vi "Read RT Variables.vi"(8 "error in (no error)":errorcluster, 11 "functionbase in":refnum<class "functionbase.lvclass">) -> (0 "error out":errorcluster, 2 "RT Variables.lvclass":refnum<class "RT Variables.lvclass">, 3 "functionbase out":refnum<class "functionbase.lvclass">)   [LabVIEW 2019, in "LSL.lvlib" / "functionbase.lvclass"]
uses:
  functionbase.lvclass
  variables/RT Variables/RT Variables.lvclass
  functionbase.lvclass/functionbase.ctl
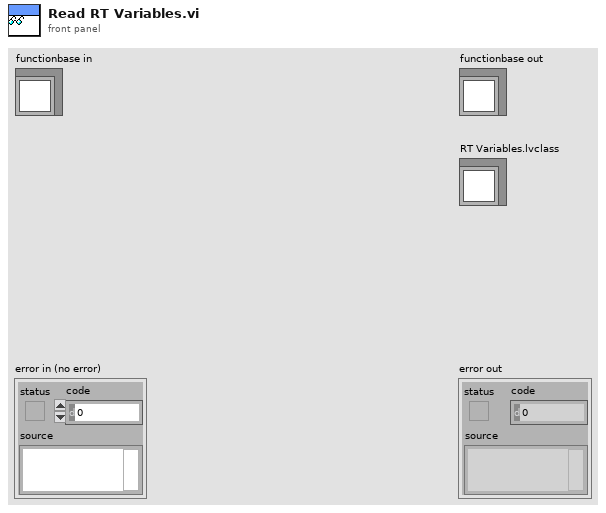
[diagram p1: front panel]
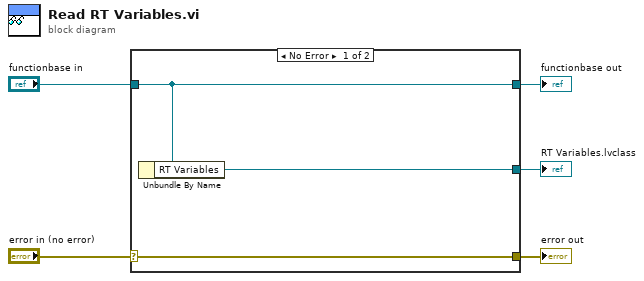
[diagram p0: block diagram]
diagram:
  n1 = case shown="No Error" "error in (no error)" {
    selector: "error in (no error)" -> [w8 w9]
    tunnel: [w8 w9] -> w4
    tunnel: [w7 w10] -> w2
    tunnel: "functionbase in" -> [w7 w10]
    tunnel: [w6 _] -> w1
    frame No Error {
      n2 = Unbundle By Name(w7) -> ("RT Variables"=w6:refnum<class "RT Variables.lvclass">)
    }
    frame Error {
    }
  }
  "error out" <- w4
  "functionbase out" <- w2
  "RT Variables.lvclass" <- w1
